vi "Joystick Commands.vi"   [LabVIEW 2016]
uses:
  <vilib>/Rock Robotics/WPI/Utilities/WPI_GetSetVariantRefNum.vi
  Robot Global Data.vi
  <vilib>/Rock Robotics/Network Tables/NT Write Boolean Array.vi
  <vilib>/Rock Robotics/Network Tables/NT Write Boolean.vi
  <vilib>/Rock Robotics/Network Tables/NT Write Numeric Array.vi
types:
  T1 = typedef "WPI_JoystickDevRef.ctl" = cluster{"Device":T2}
  T2 = typedef "WPI_JoystickDeviceEnum.ctl" = enum16{"USB 0", "USB 1", "USB 2", "USB 3", "USB 4", "USB 5"}
  T3 = typedef "WPI_DriverStationRobotMode2.ctl" = enum16{"Autonomous Disabled", "Autonomous Enabled", "Teleop Disabled", "Teleop Enabled", "Disconnected", "Finish", "Test Disabled", "Test Enabled", "Emergency Stopped"}
  T4 = cluster{"Buttons[0]":bool, "Buttons[1]":bool, "Buttons[2]":bool, "Buttons[3]":bool, "Buttons[4]":bool, "Buttons[5]":bool, "Buttons[6]":bool, "Buttons[7]":bool, "Buttons[8]":bool}
  T5 = cluster{"POVs[0]":i16, "POVs[1]":i16, "POVs[2]":i16, "POVs[3]":i16, "POVs[4]":i16, "POVs[5]":i16, "POVs[6]":i16, "POVs[7]":i16, "POVs[8]":i16}
  T6 = cluster{"Axes[0]":dbl, "Axes[1]":dbl, "Axes[2]":dbl, "Axes[3]":dbl, "Axes[4]":dbl, "Axes[5]":dbl, "Axes[6]":dbl, "Axes[7]":dbl, "Axes[8]":dbl}
  T7 = enum16{"Shooter 1 Speed Increase", "Shooter 1 Speed Decrease", "Shooter 2 Speed Increase", "Shooter 2 Speed Decrease", "Nothing Changed", "Set Zero"}
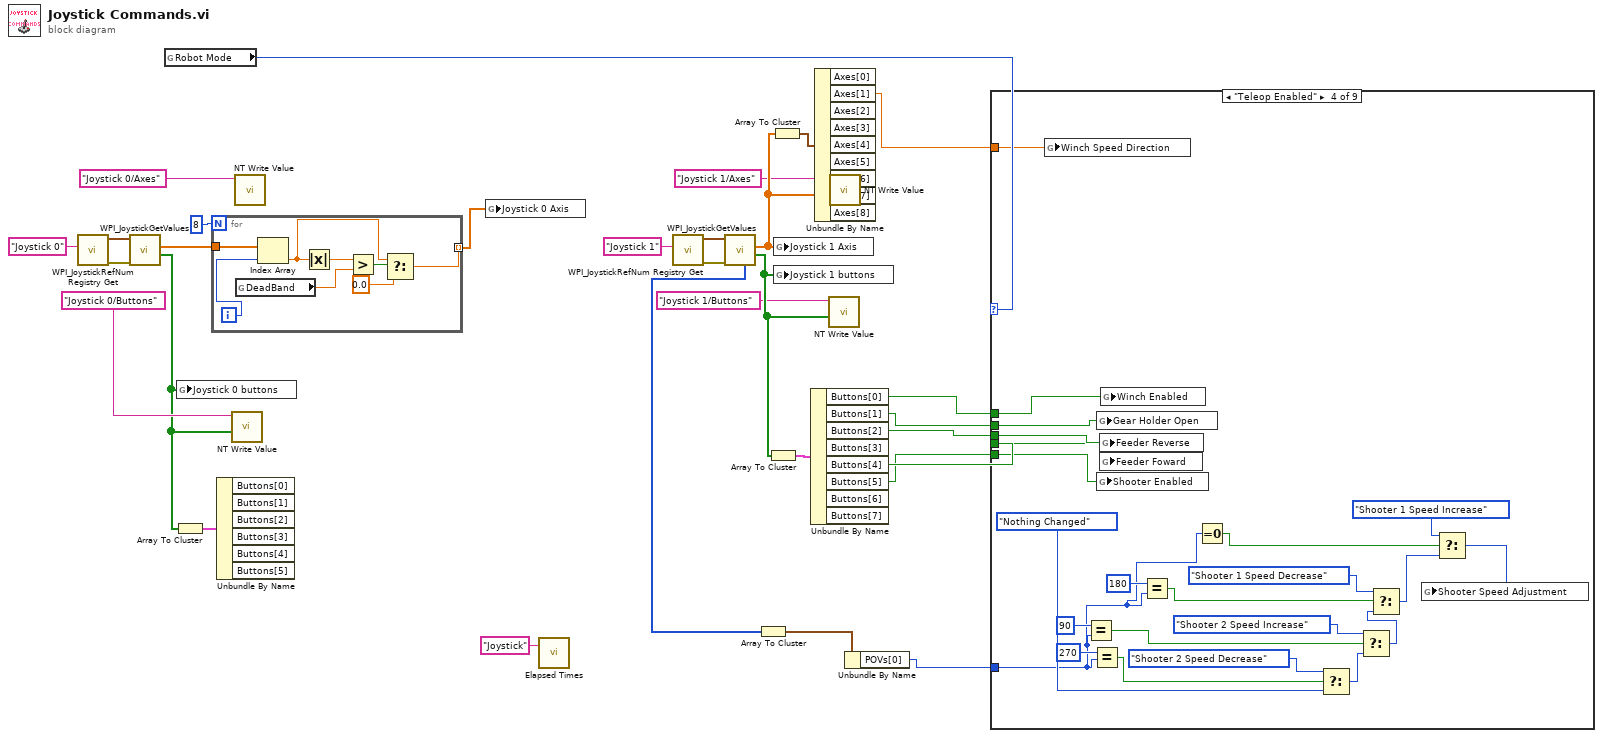
[diagram p0: block diagram]
diagram:
  n1 = call <vilib>:"WPI_JoystickRefNum Registry Get.vi"("refnum name"="Joystick 0") -> ("error out"=w27:errorcluster, "JoystickDevRef"=w28:T1)  [unwired: 1 in, 8 out]
  n2 = call <vilib>:"WPI_JoystickGetValues.vi"("error in (no error)"=w27, "JoystickDevRef"=w28) -> ("Buttons"=w14:bool[], "Axes"=w16:dbl[])  [unwired: 5 in, 3 out]
  n3 = global read "Robot Global Data.vi" "Robot Mode"() -> (w13:T3)
  n4 = Array To Cluster(array=w14) -> (cluster=w26:T4)
  n5 = global write "Robot Global Data.vi" "Joystick 0 buttons"(w14) -> ()
  n6 = for {
    N: 8 -> [_]
    tunnel: w16 -> [w38]
    tunnel: [w32] -> w2 mode=indexing
    i -> [w31]
    n7 = global read "Robot Global Data.vi" "DeadBand"() -> (w36:dbl)
    n8 = Index Array(array=w38, index=w31) -> (element=w34:dbl)
    n9 = Absolute Value(x=w34) -> (abs(x)=w37:dbl)
    n10 = Greater?(x=w37, y=w36) -> (0:w35:bool)
    n11 = Select(t=w34, s=w35, f=0.0) -> (s? t:f=w32:dbl)
  }
  n12 = Unbundle By Name(w26) -> ()  [unwired: 6 out]
  n13 = call-poly <vilib>:"NT Write Value.vi"("Boolean Array"=w14, "Name"="Joystick 0/Buttons") -> ()  [unwired: 9 in, 1 out]
  n14 = call-poly <vilib>:"NT Write Value.vi"("Name"="Joystick 0/Axes") -> ()  [unwired: 10 in, 1 out]
  n15 = global write "Robot Global Data.vi" "Joystick 0 Axis"(w2) -> ()
  n16 = call "Elapsed Times.vi"("Call Name"="Joystick") -> ()  [unwired: 2 in, 1 out]
  n17 = call <vilib>:"WPI_JoystickRefNum Registry Get.vi"("refnum name"="Joystick 1") -> ("error out"=w24:errorcluster, "JoystickDevRef"=w25:T1)  [unwired: 1 in, 8 out]
  n18 = call <vilib>:"WPI_JoystickGetValues.vi"("error in (no error)"=w24, "JoystickDevRef"=w25) -> ("Buttons"=w18:bool[], "Axes"=w20:dbl[], "POVs"=w6:i16[])  [unwired: 5 in, 2 out]
  n19 = Array To Cluster(array=w6) -> (cluster=w5:T5)
  n20 = Array To Cluster(array=w18) -> (cluster=w23:T4)
  n21 = Array To Cluster(array=w20) -> (cluster=w22:T6)
  n22 = global write "Robot Global Data.vi" "Joystick 1 Axis"(w20) -> ()
  n23 = global write "Robot Global Data.vi" "Joystick 1 buttons"(w18) -> ()
  n24 = Unbundle By Name(w23) -> ("Buttons[0]"=w11:bool, "Buttons[1]"=w8:bool, "Buttons[2]"=w9:bool, "Buttons[4]"=w10:bool, "Buttons[5]"=w7:bool)  [unwired: 3 out]
  n25 = Unbundle By Name(w22) -> ("Axes[1]"=w12:dbl)  [unwired: 8 out]
  n26 = call-poly <vilib>:"NT Write Value.vi"("Boolean Array"=w18, "Name"="Joystick 1/Buttons") -> ()  [unwired: 9 in, 1 out]
  n27 = call-poly <vilib>:"NT Write Value.vi"("Numeric Array"=w20, "Name"="Joystick 1/Axes") -> ()  [unwired: 9 in, 1 out]
  n28 = Unbundle By Name(w5) -> ("POVs[0]"=w4:i16)
  n29 = case shown="\"Teleop Enabled\"" w13 {
    tunnel: w12 -> [_ _ _ w61 _ _ _ _ _]
    tunnel: w11 -> [_ _ _ w60 _ _ _ _ _]
    tunnel: w9 -> [_ _ _ w59 _ _ _ _ _]
    tunnel: w10 -> [_ _ _ w58 _ _ _ _ _]
    tunnel: w8 -> [_ _ _ w57 _ _ _ _ _]
    tunnel: w7 -> [_ _ _ w56 _ _ _ _ _]
    tunnel: w4 -> [_ _ _ w39 _ _ _ _ _]
    frame "Autonomous Disabled", Default {
    }
    frame "Autonomous Enabled" {
    }
    frame "Teleop Disabled" {
    }
    frame "Teleop Enabled" {
      n30 = global write "Robot Global Data.vi" "Winch Speed Direction"(w61) -> ()
      n31 = Equal?(x=i16 90, y=w39) -> (x = y?=w44:bool)
      n32 = Equal?(x=i16 270, y=w39) -> (x = y?=w43:bool)
      n33 = global write "Robot Global Data.vi" "Gear Holder Open"(w57) -> ()
      n34 = global write "Robot Global Data.vi" "Shooter Enabled"(w56) -> ()
      n35 = global write "Robot Global Data.vi" "Feeder Reverse"(w59) -> ()
      n36 = global write "Robot Global Data.vi" "Feeder Foward"(w58) -> ()
      n37 = global write "Robot Global Data.vi" "Winch Enabled"(w60) -> ()
      n38 = Equal?(x=i16 180, y=w39) -> (x = y?=w45:bool)
      n39 = Equal To 0?(x=w39) -> (x = 0?=w46:bool)
      n40 = Select(t=T7."Shooter 2 Speed Decrease" ("Shooter Speed Adjustment"), s=w43, f=T7."Nothing Changed" ("Shooter Speed Adjustment")) -> (s? t:f=w50:T7)
      n41 = Select(t=T7."Shooter 2 Speed Increase" ("Shooter Speed Adjustment"), s=w44, f=w50) -> (s? t:f=w49:T7)
      n42 = Select(t=T7."Shooter 1 Speed Decrease" ("Shooter Speed Adjustment"), s=w45, f=w49) -> (s? t:f=w48:T7)
      n43 = Select(t=T7."Shooter 1 Speed Increase" ("Shooter Speed Adjustment"), s=w46, f=w48) -> (s? t:f=w47:T7)
      n44 = global write "Robot Global Data.vi" "Shooter Speed Adjustment"(w47) -> ()
    }
    frame "Disconnected" {
    }
    frame "Finish" {
    }
    frame "Test Disabled" {
    }
    frame "Test Enabled" {
    }
    frame "Emergency Stopped" {
    }
  }
